vi "OdorSystem-counter-V1.1.vi"() -> ()   [LabVIEW 2019]
doc: "Synchronize Correlated Digital Output with Analog Input Using NI-DAQmx \n\nOverview:\nThis example uses DAQmx to synchronize finite generation and acquisition of Correlated Digital Output with an Analog Input Task respectively.\n\nDescriptions:\nCorrelated I/O enables synchronization of on board digital I/O lines to a clock reference. Digital and Analog samples can be synchronized in time by sharing the AI clock as the source of your digital I/O clock. You may also use the Counter Output pulse as the Source of Digital Timing. Hence, set the Source for Digital Timing as ai/SampleClock.This example will work on any device that uses DAQmx and supports Correlated Digital I/O. To perform Correlated Digital I/O on 9172 Chassis, you need a Correlated Module in slot 1-4 of the chassis. \n\nRequirements:\n1. LabVIEW 2012 or compatible.\n2. NI-DAQmx 15.5.1 or compatible.\n\nInstructions:\n1. Set all the control values on the front panel corresponding to the physical channel to be used on the DAQ device.\n2. Run this VI.\n3. Monitor the analog input voltage measured and ramp signal generated from specified channels. \n\nBlock Diagram Steps:\n1. Creates channels to measure voltage and to generate digital signals \n2. Sets the source of the Sample Clock, the rate of the Sample Clock, and the number of samples to acquire or generate.\n3. Generates an array containing a ramp pattern and write to digital output lines.\n4. Transitions the tasks to running state to begin measuring and generating data.\n5. Reads the waveform from the analog input channel and waits for the digital output generation to complete.\n6. Clears the tasks.\n7. Displays any error occurs."
uses:
  StatesEnum.ctl
  <vilib>/DAQmx/write.llb/DAQmx Write (Digital 1D Bool NChan 1Samp 1Line).vi
  <vilib>/DAQmx/write.llb/DAQmx Write (Digital Wfm 1Chan NSamp).vi
  <vilib>/DAQmx/miscellaneous.llb/DAQmx Fill In Error Info.vi
  <vilib>/DAQmx/create/channels.llb/DAQmx Create Channel (CO-Pulse Generation-Frequency).vi
  <vilib>/Waveform/DWDTOps.llb/Digital Pattern Generator (Single Value).vi
  <vilib>/Waveform/DWDTOps.llb/DWDT Append Digital Samples.vi
  <vilib>/DAQmx/configure/timing.llb/DAQmx Timing (Implicit).vi
  <vilib>/Waveform/DWDTOps.llb/DWDT Append Digital Signals.vi
  <vilib>/Waveform/DWDTOps.llb/DWDT Digital to Boolean Array.vi
  <vilib>/DAQmx/create/channels.llb/DAQmx Create Channel (DO-Digital Output).vi
  <vilib>/DAQmx/configure/timing.llb/DAQmx Timing (Sample Clock).vi
  <vilib>/Waveform/DWDTOps.llb/DWDT Uncompress Digital.vi
panel:
  in  "Use Default vavle":bool=TRUE
  in  "Selected default valve":u8(knob)=8 min=1 max=8 step=1 scale=1.0..8.0
  out "Experiment running":bool
  out "State":T1
  in  "Select experiment":enum32{"Single trial", "Trial series"}(tab)
  out "Time elapsed":dbl format="%.1f"
  in  "Start single trial":bool
  out "single trial done":bool
  in  "Select valve":u8(knob)=1 min=1 max=8 step=1 scale=1.0..8.0
  out "Pause elapsed time":dbl format="%#.1f"
  out "In between trials":bool
  out "Trial elapsed time":dbl format="%.1f"
  out "Total elapsed time":dbl format="%.1f"
  out "Estimated total time":dbl
  out "Current list index":i32
  out "Current Valve":u8
  in  "Time between trials":u16=10 min=1 max=900 step=1
  in  "Start trial series":bool
  in  "Valve order list":i8[](array[numeric]) min=1 max=8 step=1
  out "Digitaler output":digitalwaveform(graph)
  out "Stop Boolesch":bool
  in  "Total trial time":dbl=20.0 min=1.0 step=0.1
  in  "Valve opening Time":dbl=10.0 min=0.0 step=0.1
  in  "Valve delay":dbl=2.0 min=0.0 step=0.1
  in  "Stopp":bool
  out "Digital Waveform Graph":digitalwaveform(graph)
  # "All times are in second!"
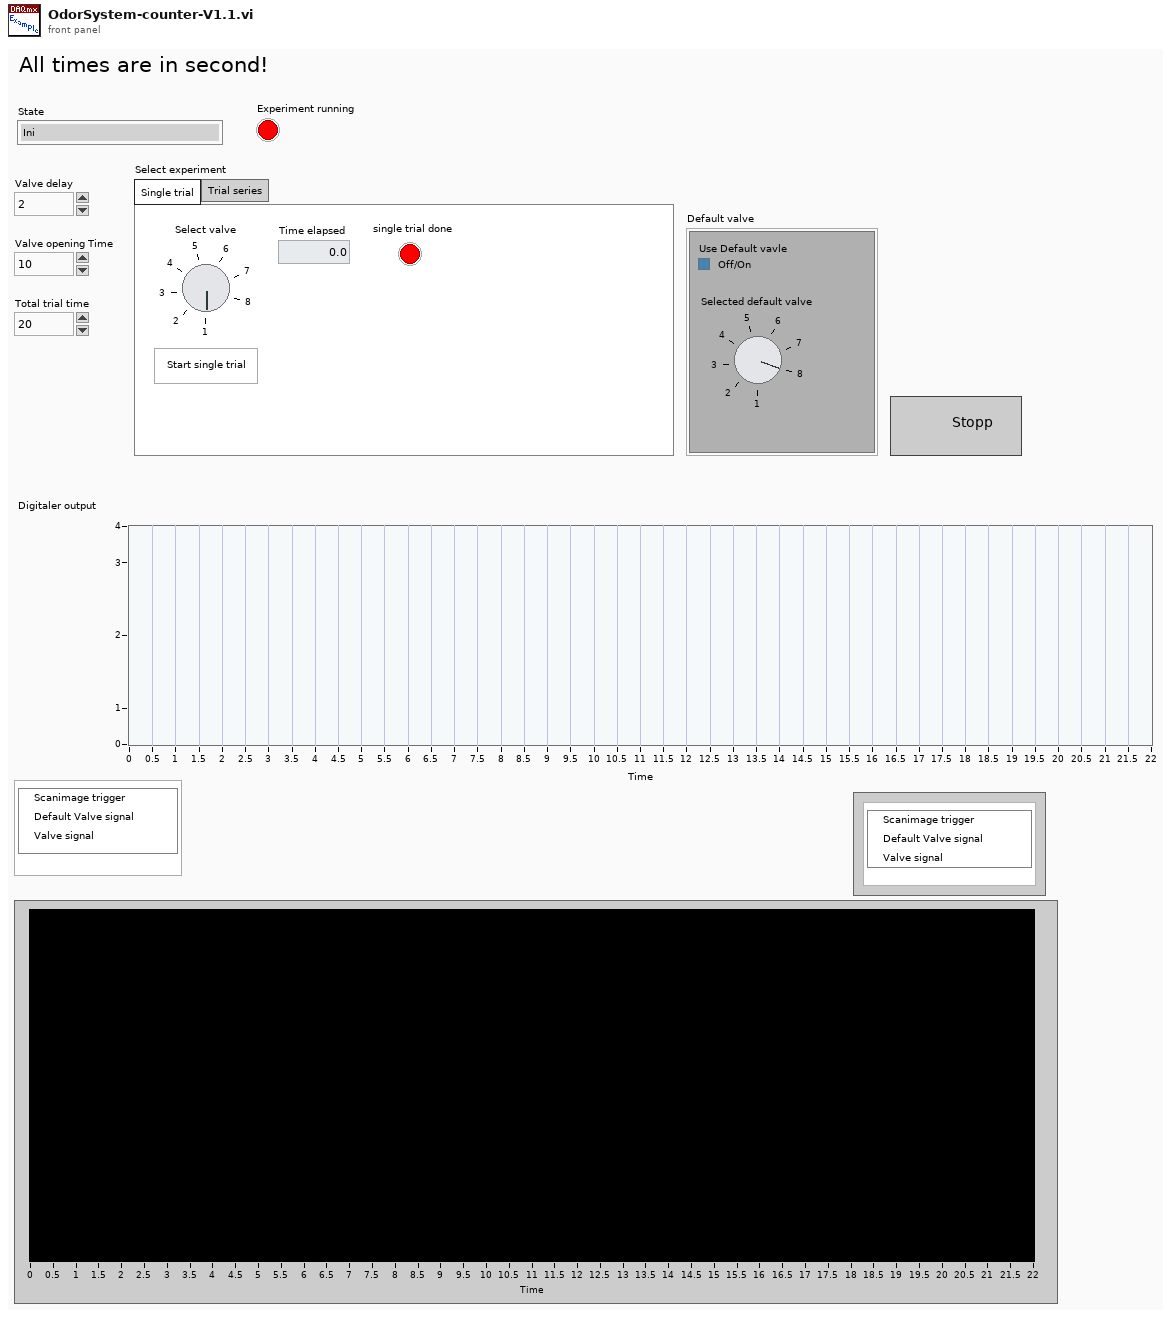
[diagram p1: front panel]
types:
  T1 = typedef "StatesEnum.ctl" = enum16{"Ini", "Standby", "Start Trial", "Start trial series", "Stop"}
  T2 = enum8{"Enabled", "Disabled", "Disabled and Grayed Out"}
  T3 = enum32{"Page Enabled", "Page Disabled", "Page Disabled & Grayed"}
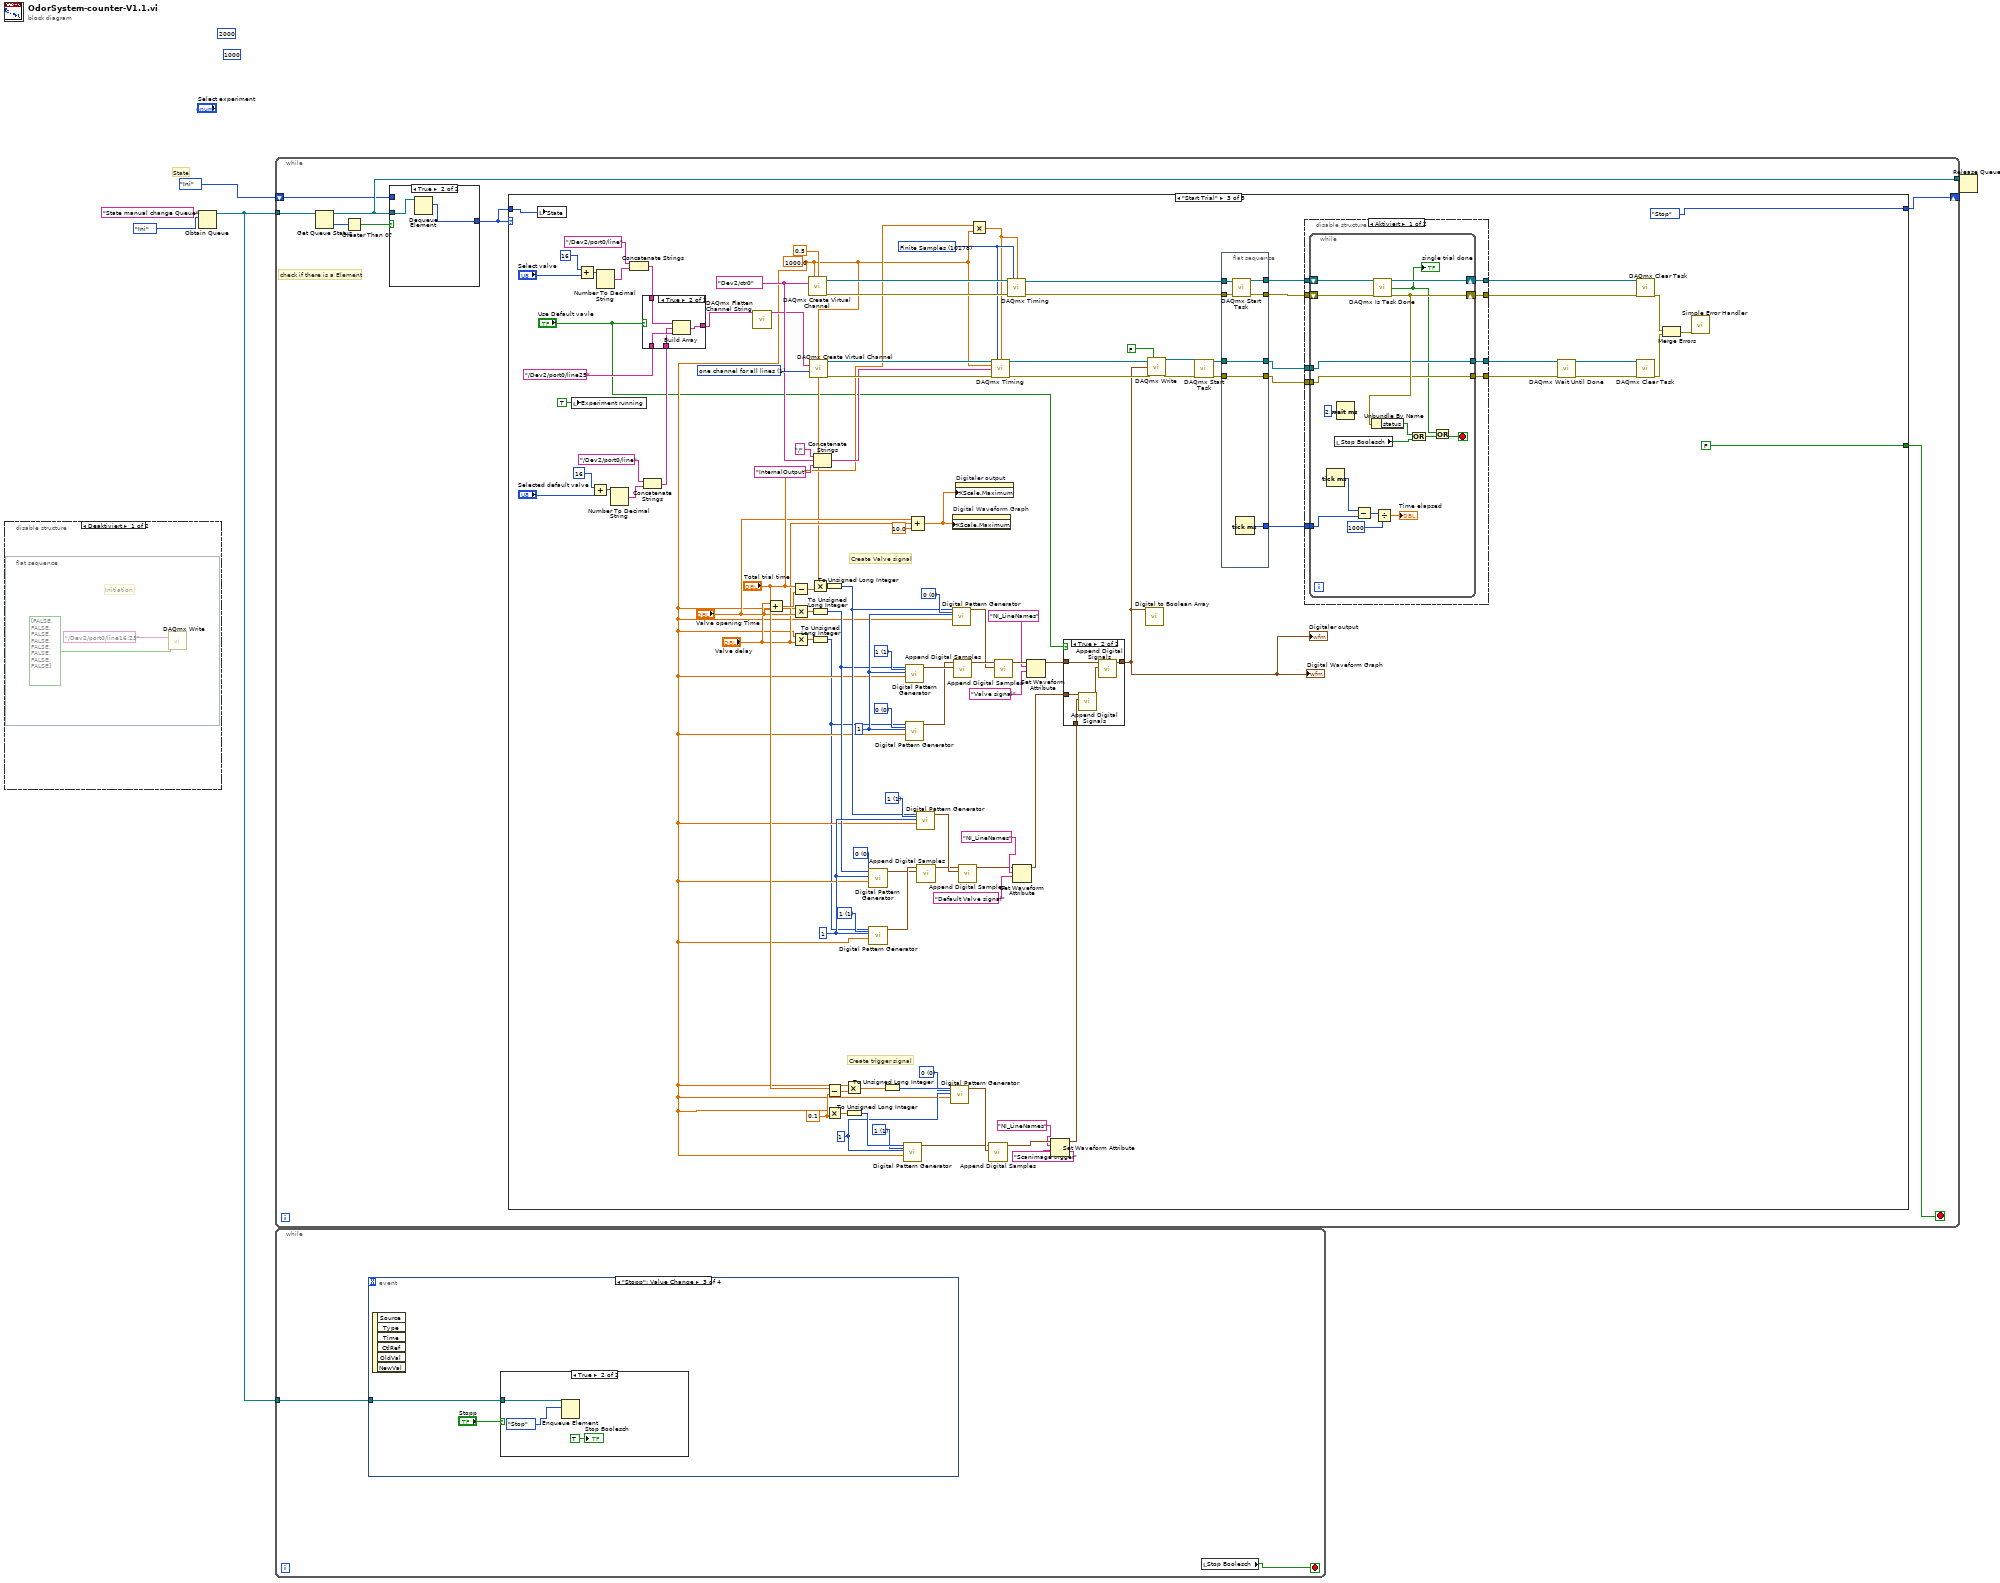
[diagram p0: block diagram]
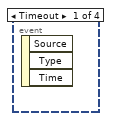
[diagram p3: hidden frame]
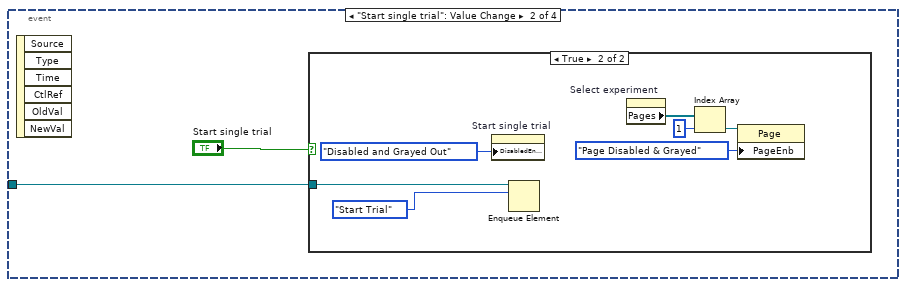
[diagram p4: hidden frame]
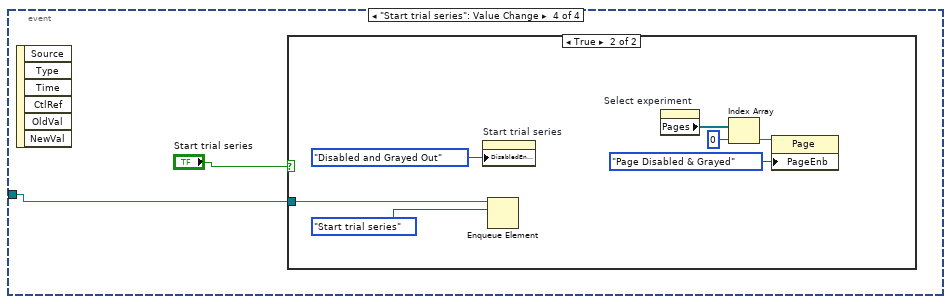
[diagram p7: hidden frame]
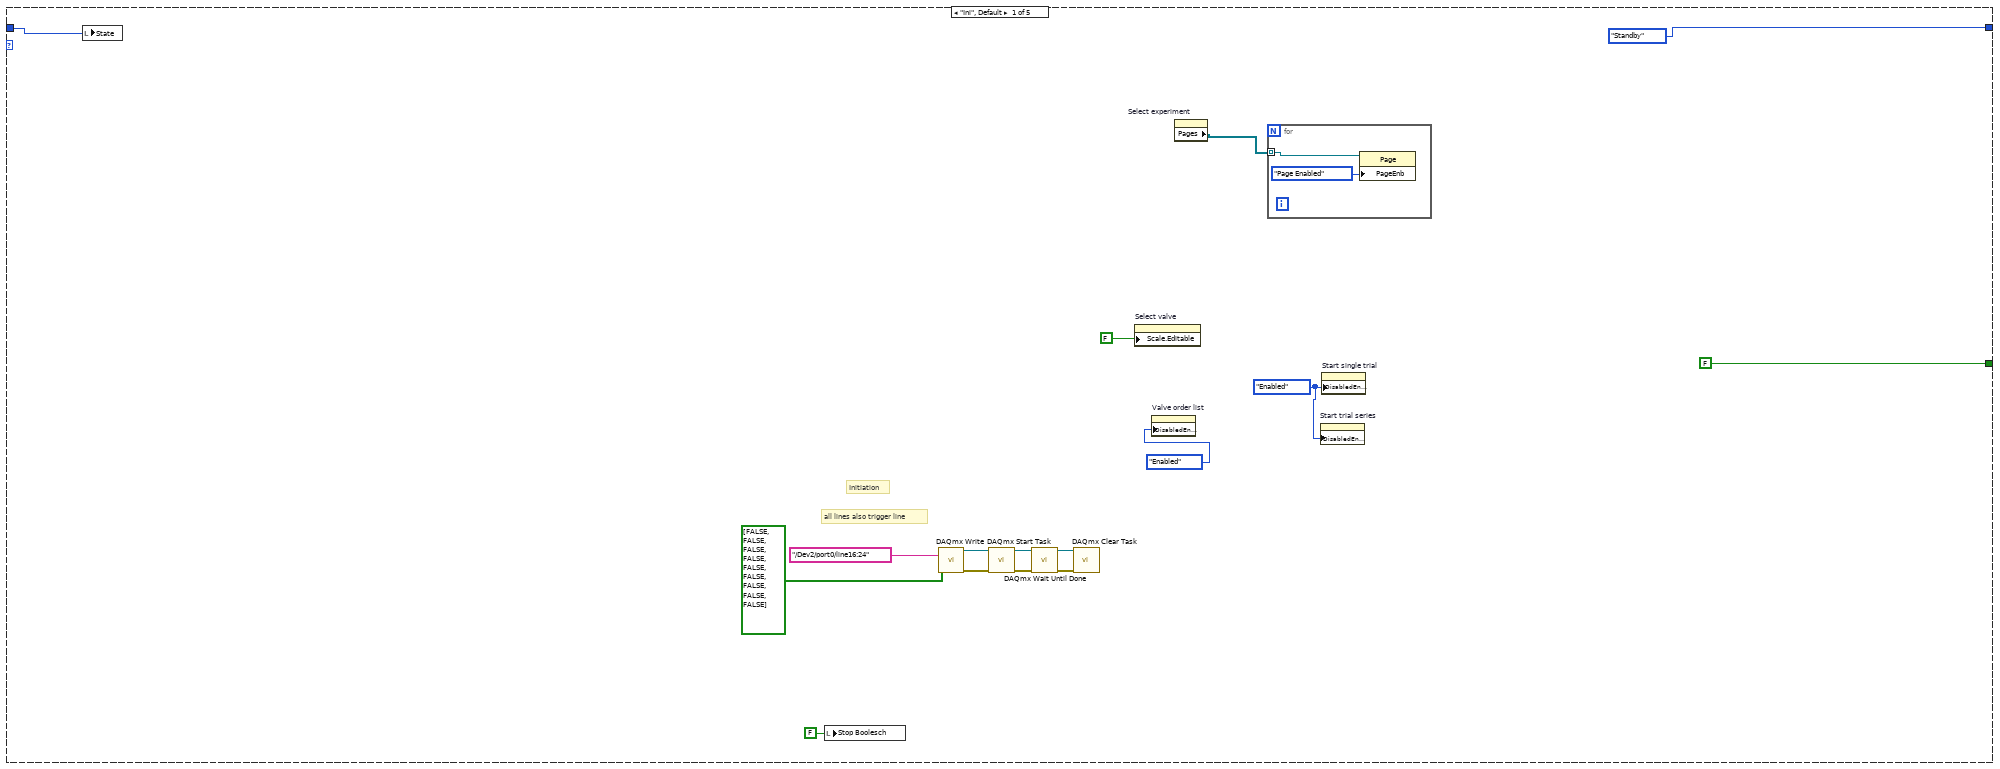
[diagram p10: hidden frame]
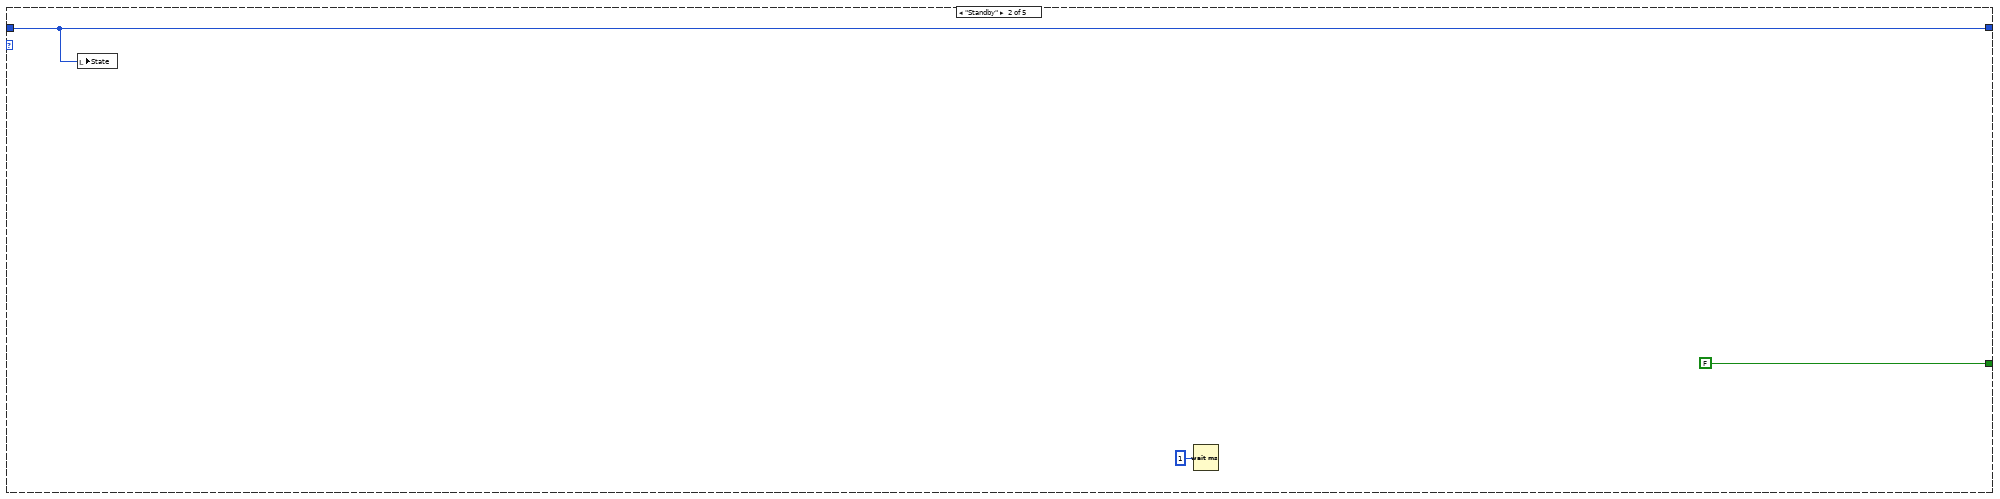
[diagram p11: hidden frame]
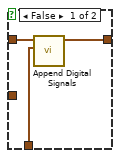
[diagram p12: hidden frame]
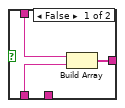
[diagram p13: hidden frame]
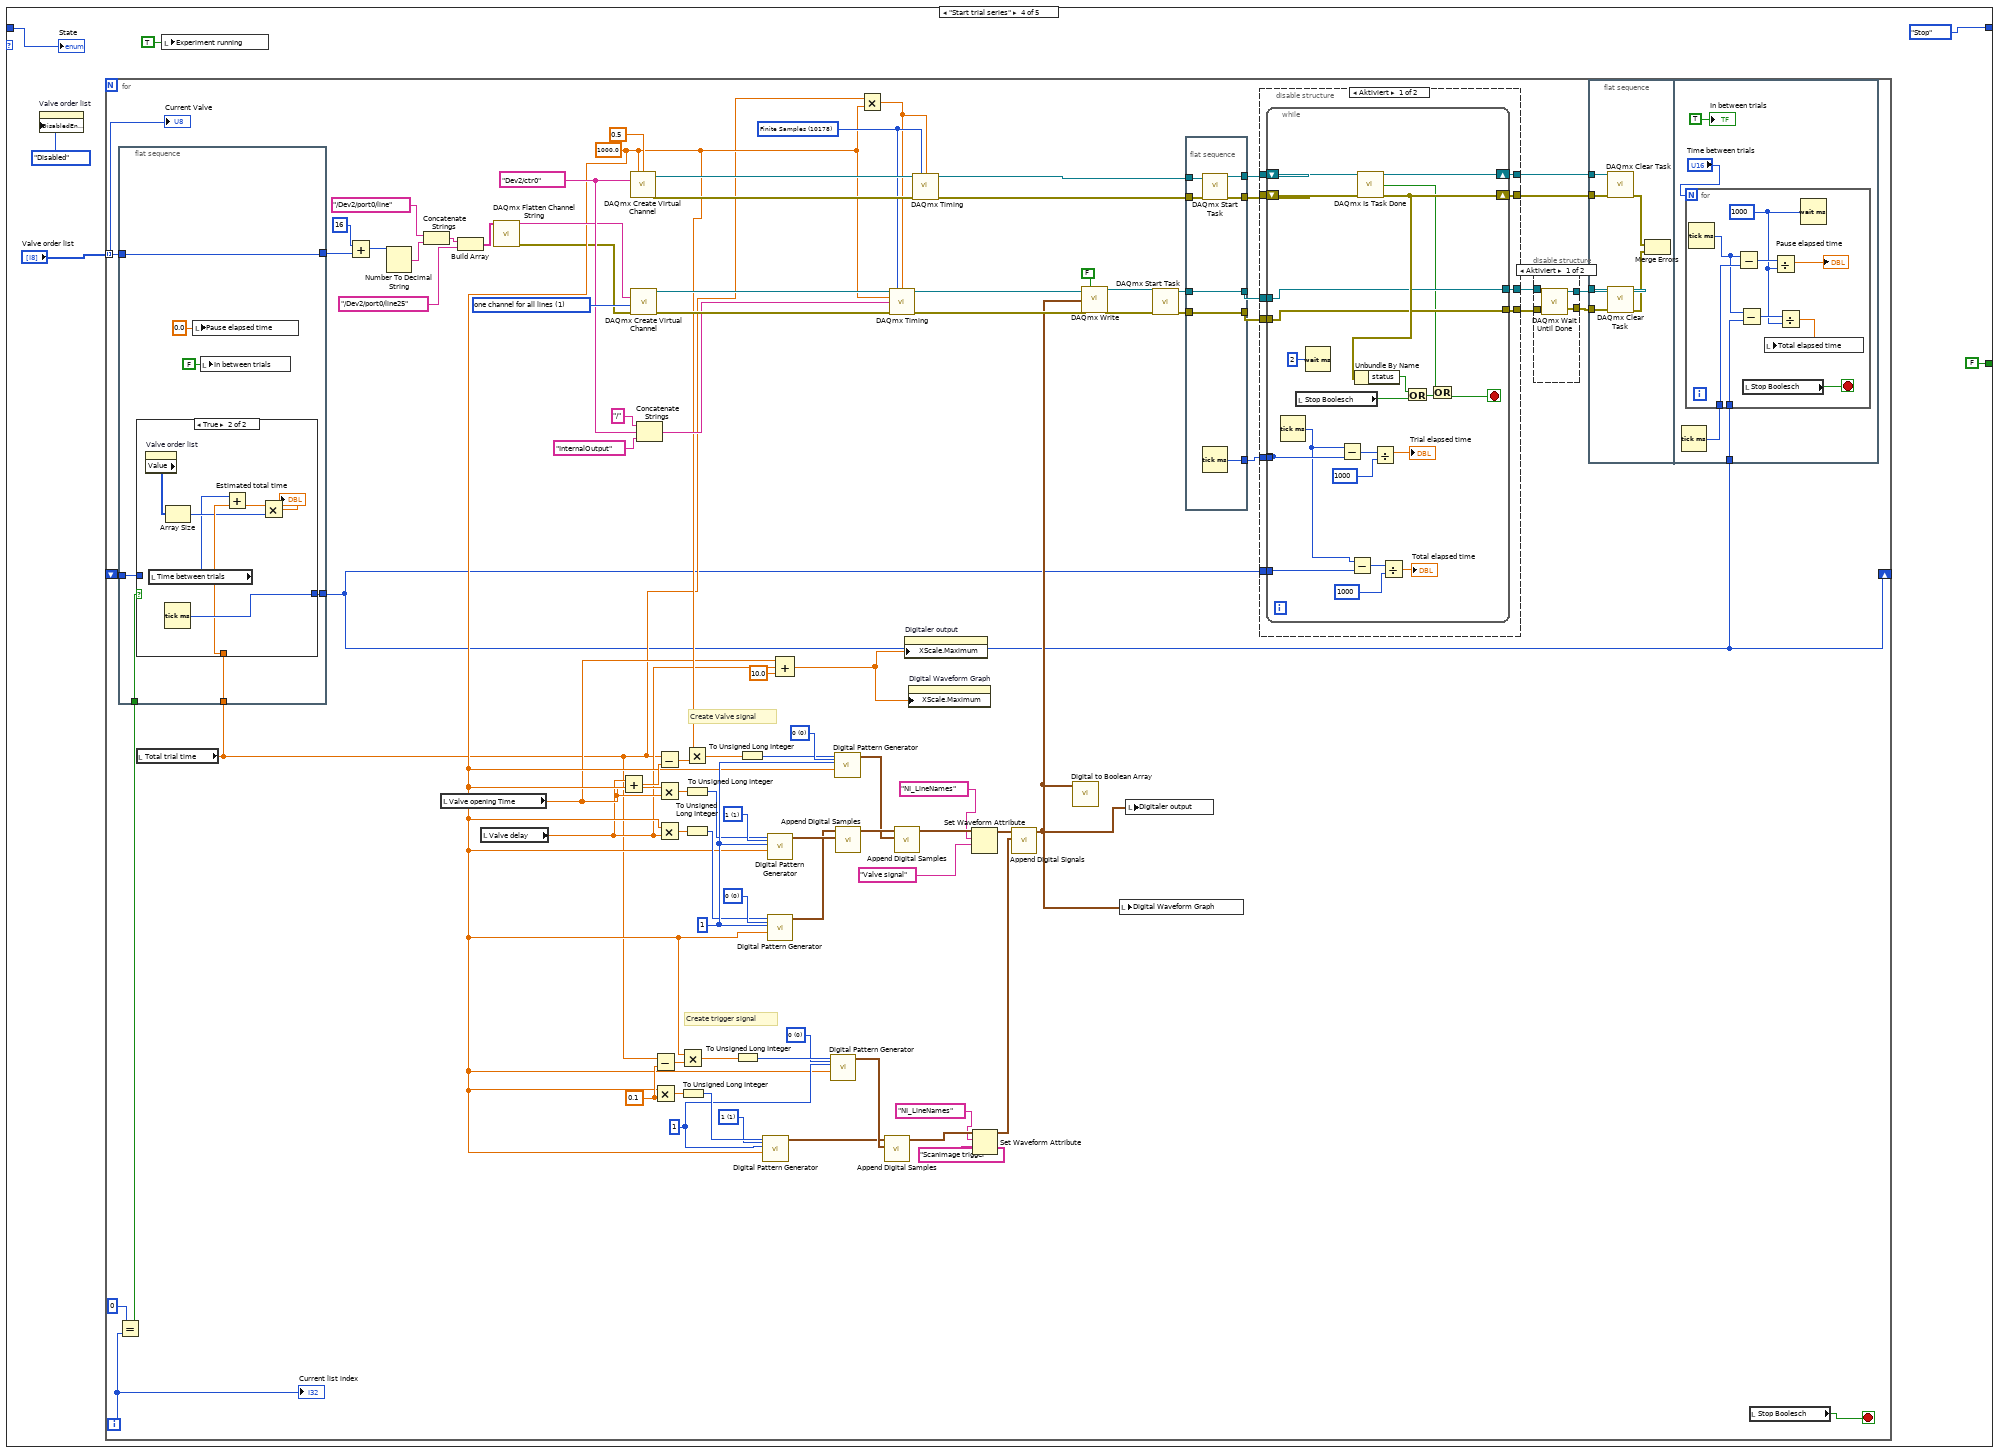
[diagram p15: hidden frame]
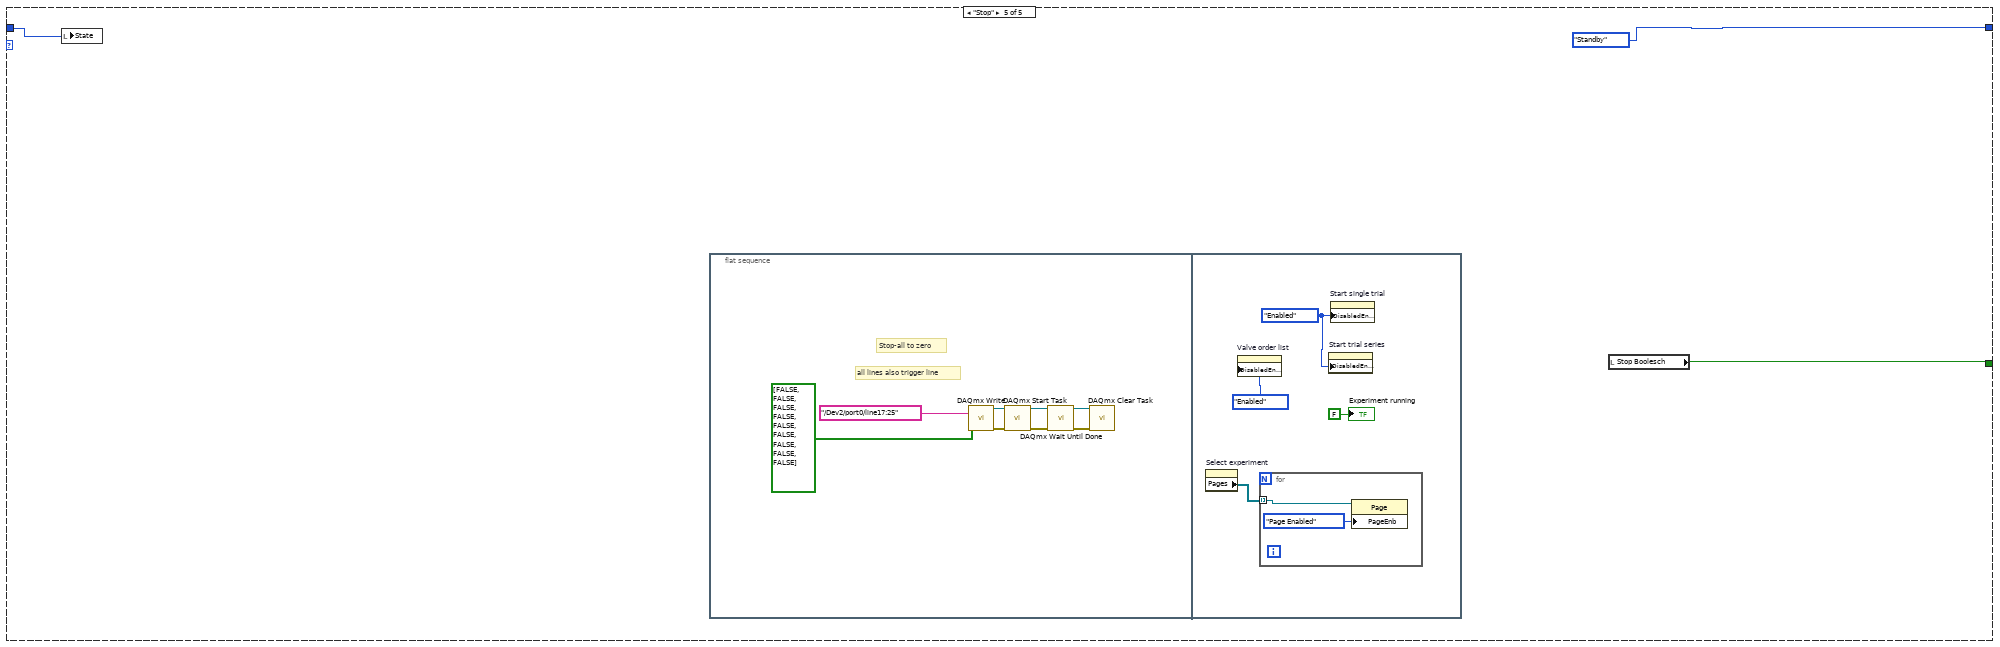
[diagram p19: hidden frame]
diagram:
  (unwired) u32 2000 ("number of samples")
  (unwired) u32 1000 ("number of samples")
  # "State"
  n1 = disable-structure shown="Deaktiviert" {
    frame Disabled {
      n2 = flat-sequence {
        frame #0 {
          # "Initiation"
          n3 = call-poly <vilib>:"DAQmx Write.vi"("task/channels in"="/Dev2/port0/line16:23" ("string"), "data"=bool[] [FALSE, FALSE, FALSE, FALSE, FALSE, FALSE, FALSE, FALSE]) -> ()  [unwired: 11 in, 3 out]
        }
      }
    }
    frame Enabled {
    }
  }
  n4 = Obtain Queue(name (unnamed)="State manual change Queue", element data type=StatesEnum."Ini" ("Enum")) -> (queue out=w4:refnum<queue>)  [unwired: 3 in, 2 out]
  n5 = while {
    tunnel: w4 -> [w13]
    tunnel: [w12] -> w3
    shift-right: [w8] -> _
    shift-left: StatesEnum."Ini" -> [w9]
    stop <- w11 stop-if-true
    # "check if there is a Element"
    n6 = Get Queue Status(queue=w13) -> (queue out=w12:refnum<queue>, # elements in queue=w15:i32)  [unwired: 2 in, 6 out]
    n7 = Greater Than 0?(x=w15) -> (x > 0?=w14:bool)
    n8 = case shown="True" w14 {
      tunnel: w12 -> [_ w18]
      tunnel: w9 -> [w16 _]
      tunnel: [w16 w17] -> w10
      frame False {
      }
      frame True {
        n9 = Dequeue Element(queue=w18) -> (element=w17:T1)  [unwired: 2 in, 3 out]
      }
    }
    n10 = case shown="\"Start Trial\"" w10 {
      tunnel: w10 -> [w29 w37 w66 w199 w369]
      tunnel: [FALSE ("Stop Boolesch") FALSE ("Stop Boolesch") FALSE ("Stop Boolesch") FALSE ("Stop Boolesch") w371] -> w11
      tunnel: [StatesEnum."Standby" ("Enum") w37 StatesEnum."Stop" ("Enum") StatesEnum."Stop" ("Enum") StatesEnum."Standby" ("Enum")] -> w8
      frame "Ini", Default {
        w22 = T2."Enabled" ("Deaktiviert")
        # "all lines also trigger line"
        # "Initiation"
        n11 = local write "State"(w29) -> ()
        n12 = local write "Stop Boolesch"(FALSE ("Stop Boolesch")) -> ()
        n13 = call-poly <vilib>:"DAQmx Write.vi"("task/channels in"="/Dev2/port0/line16:24" ("string"), "data"=bool[] [FALSE, FALSE, FALSE, FALSE, FALSE, FALSE, FALSE, FALSE, FALSE]) -> ("task out"=w24:refnum<k21>, "error out"=w23:errorcluster)  [unwired: 11 in, 1 out]
        n14 = call <vilib>:"DAQmx Start Task.vi"("task/channels in"=w24, "error in"=w23) -> ("task out"=w28:refnum<k21>, "error out"=w26:errorcluster)  [unwired: 12 in]
        n15 = call <vilib>:"DAQmx Wait Until Done.vi"("task/channels in"=w28, "error in"=w26) -> ("task out"=w27:refnum<k21>, "error out"=w25:errorcluster)  [unwired: 12 in]
        n16 = call <vilib>:"DAQmx Clear Task.vi"("task in"=w27, "error in"=w25) -> ()  [unwired: 13 in, 1 out]
        n17 = property on="Select valve" class="Knob (strict)"("Scale.Editable"=FALSE ("Skala.Editierbar")) -> ()  [unwired: 2 in, 2 out]
        n18 = property on="Valve order list" class="Arr (strict)"("DisabledEnum"=T2."Enabled" ("Deaktiviert")) -> ()  [unwired: 2 in, 2 out]
        n19 = property on="Select experiment" class="TabCtl (strict)"() -> ("Pages"=w20:refnum<vi>[])  [unwired: 2 in, 2 out]
        n20 = for {
          tunnel: w20 -> [w35] mode=indexing
          n21 = property class="Page"(reference=w35, "PageEnb"=T3."Page Enabled" ("Aktiv-Status der Seite")) -> ()  [unwired: 1 in, 2 out]
        }
        n22 = property on="Start trial series" class="Bool"("DisabledEnum"=w22) -> ()  [unwired: 2 in, 2 out]
        n23 = property on="Start single trial" class="Bool"("DisabledEnum"=w22) -> ()  [unwired: 2 in, 2 out]
      }
      frame "Standby" {
        n24 = local write "State"(w37) -> ()
        n25 = Wait (ms)(milliseconds to wait=u32 1 ("Zu wartende ms")) -> ()  [unwired: 1 out]
      }
      frame "Start Trial" {
        w52 = u32 1 ("number of signals")
        w55 = u8 1 items=["0", "1", "Z", "L", "H", "X", "T", "V"] ("value")
        w54 = u8 0 items=["0", "1", "Z", "L", "H", "X", "T", "V"] ("value")
        w53 = u8 1 items=["0", "1", "Z", "L", "H", "X", "T", "V"] ("value")
        w89 = 0.1 ("y")
        w96 = u32 1 ("number of signals")
        w98 = u8 0 items=["0", "1", "Z", "L", "H", "X", "T", "V"] ("value")
        w97 = u8 1 items=["0", "1", "Z", "L", "H", "X", "T", "V"] ("value")
        w114 = tag "Dev2/ctr0" ("counter")
        w49 = 1000.0 ("frequency")
        w123 = u32 1 ("number of signals")
        w124 = u8 0 items=["0", "1", "Z", "L", "H", "X", "T", "V"] ("value")
        w125 = u8 1 items=["0", "1", "Z", "L", "H", "X", "T", "V"] ("value")
        w126 = u8 0 items=["0", "1", "Z", "L", "H", "X", "T", "V"] ("value")
        w137 = 1 items=["one channel for each line", "one channel for all lines"] ("line grouping")
        w118 = 10178 items=["Finite Samples"=10178, "Continuous Samples"=10123] ("sample mode")
        # "Create trigger signal"
        # "Create Valve signal"
        n26 = local write "State"(w66) -> ()
        n27 = local write "Experiment running"(TRUE ("Experiment running")) -> ()
        n28 = Add(x=i8 16, y="Select valve") -> (x+y=w105:u8)
        n29 = Add(x=i8 16, y="Selected default valve") -> (x+y=w46:u8)
        n30 = Number To Decimal String(number=w105) -> (decimal integer string=w106:string)  [unwired: 1 in]
        n31 = Number To Decimal String(number=w46) -> (decimal integer string=w45:string)  [unwired: 1 in]
        n32 = Concatenate Strings("/Dev2/port0/line" ("string"), w106) -> (w95:string)
        n33 = Concatenate Strings("/Dev2/port0/line" ("string"), w45) -> (w43:string)
        n34 = case shown="True" "Use Default vavle" {
          tunnel: w95 -> [w158 w161]
          tunnel: "/Dev2/port0/line25" ("string") -> [w157 w160]
          tunnel: [w156 w162] -> w93
          tunnel: w43 -> [_ w159]
          frame False {
            n35 = Build Array(w158, w157) -> (w156:string[])
          }
          frame True {
            n36 = Build Array(w161, w159, w160) -> (w162:string[])
          }
        }
        n37 = call <vilib>:"DAQmx Flatten Channel String.vi"("names in"=w93) -> ("names out"=w92:string)  [unwired: 13 in, 1 out]
        n38 = Add(x="Valve delay", y="Valve opening Time") -> (x+y=w109:dbl)
        n39 = Subtract(x="Total trial time", y=w109) -> (x-y=w108:dbl)
        n40 = Multiply(x=w49, y="Valve opening Time") -> (x*y=w111:dbl)
        n41 = Multiply(x=w49, y="Valve delay") -> (x*y=w112:dbl)
        n42 = call-poly <vilib>:"DAQmx Create Virtual Channel.vi"("frequency"=w49, "duty cycle"=0.5, "counter"=w114) -> ("task out"=w142:refnum<k21>, "error out"=w143:errorcluster)  [unwired: 11 in]
        n43 = call-poly <vilib>:"DAQmx Create Virtual Channel.vi"("lines"=w92, "line grouping"=w137) -> ("task out"=w147:refnum<k21>, "error out"=w146:errorcluster)  [unwired: 12 in]
        n44 = Multiply(x=w49, y=w108) -> (x*y=w110:dbl)
        n45 = To Unsigned Long Integer(number=w111) -> (unsigned 32bit integer=w50:u32)
        n46 = To Unsigned Long Integer(number=w112) -> (unsigned 32bit integer=w48:u32)
        n47 = Concatenate Strings("/", w114, "InternalOutput" ("string")) -> (w113:string)
        n48 = To Unsigned Long Integer(number=w110) -> (unsigned 32bit integer=w51:u32)
        n49 = Subtract(x="Total trial time", y=w89) -> (x-y=w103:dbl)
        n50 = Multiply(x=w49, y=w89) -> (x*y=w99:dbl)
        n51 = Multiply(x=w49, y=w103) -> (x*y=w101:dbl)
        n52 = To Unsigned Long Integer(number=w99) -> (unsigned 32bit integer=w100:u32)
        n53 = call-poly <vilib>:"Digital Pattern Generator.vi"("value"=w54, "sample rate"=w49, "number of signals"=w52, "number of samples"=w50) -> ("digital waveform"=w59:digitalwaveform)  [unwired: 6 in, 1 out]
        n54 = call-poly <vilib>:"Digital Pattern Generator.vi"("value"=w53, "sample rate"=w49, "number of signals"=w52, "number of samples"=w48) -> ("digital waveform"=w60:digitalwaveform)  [unwired: 6 in, 1 out]
        n55 = To Unsigned Long Integer(number=w101) -> (unsigned 32bit integer=w102:u32)
        n56 = call-poly <vilib>:"Digital Pattern Generator.vi"("value"=w97, "sample rate"=w49, "number of signals"=w96, "number of samples"=w100) -> ("digital waveform"=w77:digitalwaveform)  [unwired: 6 in, 1 out]
        n57 = call-poly <vilib>:"Digital Pattern Generator.vi"("value"=w125, "sample rate"=w49, "number of signals"=w123, "number of samples"=w50) -> ("digital waveform"=w82:digitalwaveform)  [unwired: 6 in, 1 out]
        n58 = call-poly <vilib>:"Digital Pattern Generator.vi"("value"=w126, "sample rate"=w49, "number of signals"=w123, "number of samples"=w48) -> ("digital waveform"=w81:digitalwaveform)  [unwired: 6 in, 1 out]
        n59 = Compound Arithmetic op=ADD("Valve opening Time", "Valve delay", 10.0 ("Wert")) -> (w67:dbl)
        n60 = call-poly <vilib>:"Digital Pattern Generator.vi"("value"=w55, "sample rate"=w49, "number of signals"=w52, "number of samples"=w51) -> ("digital waveform"=w62:digitalwaveform)  [unwired: 6 in, 1 out]
        n61 = call-poly <vilib>:"Append Digital Samples.vi"("digital waveform B"=w59, "digital waveform A"=w60) -> ("digital waveform out"=w61:digitalwaveform)  [unwired: 8 in, 1 out]
        n62 = call-poly <vilib>:"Digital Pattern Generator.vi"("value"=w98, "sample rate"=w49, "number of signals"=w96, "number of samples"=w102) -> ("digital waveform"=w78:digitalwaveform)  [unwired: 6 in, 1 out]
        n63 = property on="Digital Waveform Graph" class="DigitalGraph (strict)"("XScale.Maximum"=w67) -> ()  [unwired: 2 in, 2 out]
        n64 = call-poly <vilib>:"Digital Pattern Generator.vi"("value"=w124, "sample rate"=w49, "number of signals"=w123, "number of samples"=w51) -> ("digital waveform"=w79:digitalwaveform)  [unwired: 6 in, 1 out]
        n65 = call-poly <vilib>:"Append Digital Samples.vi"("digital waveform B"=w82, "digital waveform A"=w81) -> ("digital waveform out"=w80:digitalwaveform)  [unwired: 8 in, 1 out]
        n66 = property on="Digitaler output" class="DigitalGraph (strict)"("XScale.Maximum"=w67) -> ()  [unwired: 2 in, 2 out]
        n67 = call-poly <vilib>:"Append Digital Samples.vi"("digital waveform B"=w62, "digital waveform A"=w61) -> ("digital waveform out"=w56:digitalwaveform)  [unwired: 8 in, 1 out]
        n68 = Multiply(x="Total trial time", y=w49) -> (x*y=w90:dbl)
        n69 = call-poly <vilib>:"Append Digital Samples.vi"("digital waveform B"=w78, "digital waveform A"=w77) -> ("digital waveform out"=w88:digitalwaveform)  [unwired: 8 in, 1 out]
        n70 = call-poly <vilib>:"DAQmx Timing.vi"("task/channels in"=w147, "sample mode"=w118, "samples per channel"=w90, "rate"=w49, "source"=w113, "error in"=w146) -> ("task out"=w134:refnum<k21>, "error out"=w133:errorcluster)  [unwired: 8 in]
        n71 = call-poly <vilib>:"Append Digital Samples.vi"("digital waveform B"=w79, "digital waveform A"=w80) -> ("digital waveform out"=w85:digitalwaveform)  [unwired: 8 in, 1 out]
        n72 = call-poly <vilib>:"DAQmx Timing.vi"("task/channels in"=w142, "sample mode"=w118, "samples per channel"=w90, "error in"=w143) -> ("task out"=w140:refnum<k21>, "error out"=w141:errorcluster)  [unwired: 10 in]
        n73 = Set Waveform Attribute(5:"Default Valve signal", 6:"NI_LineNames" ("name"), 7:w56) -> (3:w40:digitalwaveform)  [unwired: 1 in, 2 out]
        n74 = Set Waveform Attribute(5:"Valve signal", 6:"NI_LineNames" ("name"), 7:w85) -> (3:w76:digitalwaveform)  [unwired: 1 in, 2 out]
        n75 = Set Waveform Attribute(5:"Scanimage trigger", 6:"NI_LineNames" ("name"), 7:w88) -> (3:w75:digitalwaveform)  [unwired: 1 in, 2 out]
        n76 = case shown="True" "Use Default vavle" {
          tunnel: w76 -> [w150 w155]
          tunnel: w75 -> [w149 w153]
          tunnel: [w148 w154] -> w69
          tunnel: w40 -> [_ w152]
          frame False {
            n77 = call-poly <vilib>:"Append Digital Signals.vi"("digital waveform (low bits)"=w149, "digital waveform (high bits)"=w150) -> ("digital waveform out"=w148:digitalwaveform)  [unwired: 8 in, 1 out]
          }
          frame True {
            n78 = call-poly <vilib>:"Append Digital Signals.vi"("digital waveform (low bits)"=w153, "digital waveform (high bits)"=w152) -> ("digital waveform out"=w151:digitalwaveform)  [unwired: 8 in, 1 out]
            n79 = call-poly <vilib>:"Append Digital Signals.vi"("digital waveform (low bits)"=w151, "digital waveform (high bits)"=w155) -> ("digital waveform out"=w154:digitalwaveform)  [unwired: 8 in, 1 out]
          }
        }
        "Digital Waveform Graph" <- w69
        "Digitaler output" <- w69
        n80 = call-poly <vilib>:"Digital to Boolean Array.vi"("digital waveform"=w69) -> ()  [unwired: 9 in, 2 out]
        n81 = call-poly <vilib>:"DAQmx Write.vi"("task/channels in"=w134, "auto start"=FALSE, "data"=w69, "error in"=w133) -> ("task out"=w132:refnum<k21>, "error out"=w131:errorcluster)  [unwired: 9 in, 1 out]
        n82 = call <vilib>:"DAQmx Start Task.vi"("task/channels in"=w132, "error in"=w131) -> ("task out"=w136:refnum<k21>, "error out"=w135:errorcluster)  [unwired: 12 in]
        n83 = flat-sequence {
          tunnel: [w195] -> w145
          tunnel: [w194] -> w144
          tunnel: w141 -> [w193]
          tunnel: w140 -> [w192]
          tunnel: [w191] -> w122
          tunnel: w136 -> [w191]
          tunnel: [w190] -> w121
          tunnel: w135 -> [w190]
          tunnel: [w189] -> w64
          frame #0 {
            n84 = call <vilib>:"DAQmx Start Task.vi"("task/channels in"=w192, "error in"=w193) -> ("task out"=w195:refnum<k21>, "error out"=w194:errorcluster)  [unwired: 12 in]
            n85 = Tick Count (ms)() -> (millisecond timer value=w189:u32)
          }
        }
        n86 = disable-structure shown="Aktiviert" {
          disable-tunnel: w145 -> [w171 _]
          disable-tunnel: w144 -> [w170 _]
          disable-tunnel: [w169 _] -> w139
          disable-tunnel: [w168 _] -> w138
          disable-tunnel: w122 -> [w167 _]
          disable-tunnel: w121 -> [w166 _]
          disable-tunnel: [w165 _] -> w120
          disable-tunnel: [w164 _] -> w119
          disable-tunnel: w64 -> [w163 _]
          frame Enabled {
            n87 = while {
              shift-right: [w185] -> w168
              shift-left: w171 -> [w187]
              shift-right: [w184] -> w169
              shift-left: w170 -> [w186]
              tunnel: w167 -> [w183]
              tunnel: w166 -> [w182]
              tunnel: [w183] -> w165
              tunnel: [w182] -> w164
              tunnel: w163 -> [w175]
              stop <- w178 stop-if-true
              n88 = Tick Count (ms)() -> (millisecond timer value=w176:u32)
              n89 = local read "Stop Boolesch"() -> (w179:bool)
              n90 = Wait (ms)(milliseconds to wait=u32 2 ("Zu wartende ms")) -> ()  [unwired: 1 out]
              n91 = Subtract(x=w176, y=w175) -> (x-y=w174:u32)
              n92 = call <vilib>:"DAQmx Is Task Done.vi"("task/channels in"=w187, "error in"=w186) -> ("task out"=w185:refnum<k21>, "task done?"=w177:bool, "error out"=w184:errorcluster)  [unwired: 11 in]
              "single trial done" <- w177
              n93 = Unbundle By Name(w184) -> ("status"=w180:bool)
              n94 = Divide(x=w174, y=u32 1000) -> (x/y=→"Time elapsed":dbl)
              n95 = Or(x=w180, y=w179) -> (x .or. y?=w188:bool)
              n96 = Or(x=w177, y=w188) -> (x .or. y?=w178:bool)
            }
          }
          frame Disabled {
          }
        }
        n97 = call <vilib>:"DAQmx Wait Until Done.vi"("task/channels in"=w120) -> ("task out"=w71:refnum<k21>)  [unwired: 13 in, 1 out]
        n98 = call <vilib>:"DAQmx Clear Task.vi"("task in"=w138, "error in"=w139) -> ("error out"=w129:errorcluster)  [unwired: 13 in]
        n99 = call <vilib>:"DAQmx Clear Task.vi"("task in"=w71, "error in"=w119) -> ("error out"=w128:errorcluster)  [unwired: 13 in]
        n100 = Merge Errors(w129, w128) -> (w127:errorcluster)
        n101 = call <vilib>:"Simple Error Handler.vi"("error in (no error)"=w127) -> ()  [unwired: 4 in, 5 out]
      }
      frame "Start trial series" {
        n102 = property on="Valve order list" class="Arr (strict)"("DisabledEnum"=T2."Disabled" ("Deaktiviert")) -> ()  [unwired: 2 in, 2 out]
        n103 = for {
          tunnel: "Valve order list" -> [w207] mode=indexing
          shift-right: [w203] -> _
          shift-left: _ -> [w205]
          i -> [w213]
          stop <- w217 stop-if-true
          w238 = 0.1 ("y")
          w244 = u32 1 ("number of signals")
          w246 = u8 0 items=["0", "1", "Z", "L", "H", "X", "T", "V"] ("value")
          w245 = u8 1 items=["0", "1", "Z", "L", "H", "X", "T", "V"] ("value")
          w265 = tag "Dev2/ctr0" ("counter")
          w222 = 1000.0 ("frequency")
          w273 = u32 1 ("number of signals")
          w274 = u8 0 items=["0", "1", "Z", "L", "H", "X", "T", "V"] ("value")
          w275 = u8 1 items=["0", "1", "Z", "L", "H", "X", "T", "V"] ("value")
          w276 = u8 0 items=["0", "1", "Z", "L", "H", "X", "T", "V"] ("value")
          w284 = 1 items=["one channel for each line", "one channel for all lines"] ("line grouping")
          w269 = 10178 items=["Finite Samples"=10178, "Continuous Samples"=10123] ("sample mode")
          # "Create trigger signal"
          # "Create Valve signal"
          n104 = Equal?(x=0, y=w213) -> (x = y?=w206:bool)
          n105 = flat-sequence {
            tunnel: [w303] -> w208
            tunnel: w207 -> [w303]
            tunnel: w206 -> [w302]
            tunnel: w205 -> [w301]
            tunnel: w204 -> [w300]
            tunnel: [w299] -> w203
            frame #0 {
              n106 = case shown="True" w302 {
                tunnel: [w304 w311] -> w299
                tunnel: w301 -> [w304 _]
                tunnel: w300 -> [_ w310]
                frame False {
                }
                frame True {
                  n107 = property on="Valve order list" class="Arr (strict)"() -> ("Value"=w308:i8[])  [unwired: 2 in, 2 out]
                  n108 = local read "Time between trials"() -> (w305:u16)
                  n109 = Tick Count (ms)() -> (millisecond timer value=w311:u32)
                  n110 = Array Size(array=w308) -> (size(s)=w307:i32)
                  n111 = Add(x=w305, y=w310) -> (x+y=w306:dbl)
                  n112 = Multiply(x=w306, y=w307) -> (x*y=→"Estimated total time":dbl)
                }
              }
              n113 = local write "Pause elapsed time"(0.0 ("Pause elapsed time")) -> ()
              n114 = local write "In between trials"(FALSE ("In between trials")) -> ()
            }
          }
          n115 = local read "Total trial time"() -> (w204:dbl)
          n116 = Add(x=i8 16, y=w208) -> (x+y=w253:i8)
          n117 = Number To Decimal String(number=w253) -> (decimal integer string=w254:string)  [unwired: 1 in]
          n118 = Concatenate Strings("/Dev2/port0/line" ("string"), w254) -> (w243:string)
          n119 = local read "Valve opening Time"() -> (w219:dbl)
          n120 = Build Array(w243, "/Dev2/port0/line25" ("string")) -> (w241:string[])
          n121 = local read "Valve delay"() -> (w218:dbl)
          n122 = call <vilib>:"DAQmx Flatten Channel String.vi"("names in"=w241) -> ("names out"=w240:string, "error out"=w202:errorcluster)  [unwired: 13 in]
          n123 = Add(x=w218, y=w219) -> (x+y=w257:dbl)
          n124 = call-poly <vilib>:"DAQmx Create Virtual Channel.vi"("frequency"=w222, "duty cycle"=0.5, "counter"=w265) -> ("task out"=w287:refnum<k21>, "error out"=w288:errorcluster)  [unwired: 11 in]
          n125 = call-poly <vilib>:"DAQmx Create Virtual Channel.vi"("lines"=w240, "line grouping"=w284, "error in"=w202) -> ("task out"=w292:refnum<k21>, "error out"=w291:errorcluster)  [unwired: 11 in]
          n126 = Concatenate Strings("/", w265, "InternalOutput" ("string")) -> (w264:string)
          n127 = Subtract(x=w204, y=w238) -> (x-y=w251:dbl)
          n128 = Multiply(x=w222, y=w238) -> (x*y=w247:dbl)
          n129 = Subtract(x=w204, y=w257) -> (x-y=w256:dbl)
          n130 = Multiply(x=w222, y=w219) -> (x*y=w261:dbl)
          n131 = Multiply(x=w222, y=w218) -> (x*y=w263:dbl)
          n132 = Multiply(x=w222, y=w251) -> (x*y=w249:dbl)
          n133 = To Unsigned Long Integer(number=w247) -> (unsigned 32bit integer=w248:u32)
          n134 = Multiply(x=w222, y=w256) -> (x*y=w259:dbl)
          n135 = To Unsigned Long Integer(number=w261) -> (unsigned 32bit integer=w260:u32)
          n136 = To Unsigned Long Integer(number=w263) -> (unsigned 32bit integer=w262:u32)
          n137 = To Unsigned Long Integer(number=w249) -> (unsigned 32bit integer=w250:u32)
          n138 = To Unsigned Long Integer(number=w259) -> (unsigned 32bit integer=w258:u32)
          n139 = call-poly <vilib>:"Digital Pattern Generator.vi"("value"=w245, "sample rate"=w222, "number of signals"=w244, "number of samples"=w248) -> ("digital waveform"=w226:digitalwaveform)  [unwired: 6 in, 1 out]
          n140 = call-poly <vilib>:"Digital Pattern Generator.vi"("value"=w275, "sample rate"=w222, "number of signals"=w273, "number of samples"=w260) -> ("digital waveform"=w231:digitalwaveform)  [unwired: 6 in, 1 out]
          n141 = call-poly <vilib>:"Digital Pattern Generator.vi"("value"=w276, "sample rate"=w222, "number of signals"=w273, "number of samples"=w262) -> ("digital waveform"=w230:digitalwaveform)  [unwired: 6 in, 1 out]
          n142 = Compound Arithmetic op=ADD(w219, w218, 10.0 ("Wert")) -> (w220:dbl)
          n143 = call-poly <vilib>:"Digital Pattern Generator.vi"("value"=w246, "sample rate"=w222, "number of signals"=w244, "number of samples"=w250) -> ("digital waveform"=w227:digitalwaveform)  [unwired: 6 in, 1 out]
          n144 = call-poly <vilib>:"Digital Pattern Generator.vi"("value"=w274, "sample rate"=w222, "number of signals"=w273, "number of samples"=w258) -> ("digital waveform"=w228:digitalwaveform)  [unwired: 6 in, 1 out]
          n145 = call-poly <vilib>:"Append Digital Samples.vi"("digital waveform B"=w231, "digital waveform A"=w230) -> ("digital waveform out"=w229:digitalwaveform)  [unwired: 8 in, 1 out]
          n146 = Multiply(x=w204, y=w222) -> (x*y=w239:dbl)
          n147 = call-poly <vilib>:"Append Digital Samples.vi"("digital waveform B"=w227, "digital waveform A"=w226) -> ("digital waveform out"=w237:digitalwaveform)  [unwired: 8 in, 1 out]
          n148 = call-poly <vilib>:"DAQmx Timing.vi"("task/channels in"=w292, "sample mode"=w269, "samples per channel"=w239, "rate"=w222, "source"=w264, "error in"=w291) -> ("task out"=w281:refnum<k21>, "error out"=w280:errorcluster)  [unwired: 8 in]
          n149 = call-poly <vilib>:"Append Digital Samples.vi"("digital waveform B"=w228, "digital waveform A"=w229) -> ("digital waveform out"=w234:digitalwaveform)  [unwired: 8 in, 1 out]
          n150 = property on="Digitaler output" class="DigitalGraph (strict)"("XScale.Maximum"=w220) -> ()  [unwired: 2 in, 2 out]
          n151 = property on="Digital Waveform Graph" class="DigitalGraph (strict)"("XScale.Maximum"=w220) -> ()  [unwired: 2 in, 2 out]
          n152 = call-poly <vilib>:"DAQmx Timing.vi"("task/channels in"=w287, "sample mode"=w269, "samples per channel"=w239, "error in"=w288) -> ("task out"=w285:refnum<k21>, "error out"=w286:errorcluster)  [unwired: 10 in]
          n153 = Set Waveform Attribute(5:"Valve signal", 6:"NI_LineNames" ("name"), 7:w234) -> (3:w225:digitalwaveform)  [unwired: 1 in, 2 out]
          n154 = Set Waveform Attribute(5:"Scanimage trigger", 6:"NI_LineNames" ("name"), 7:w237) -> (3:w224:digitalwaveform)  [unwired: 1 in, 2 out]
          n155 = call-poly <vilib>:"Append Digital Signals.vi"("digital waveform (low bits)"=w224, "digital waveform (high bits)"=w225) -> ("digital waveform out"=w221:digitalwaveform)  [unwired: 8 in, 1 out]
          n156 = call-poly <vilib>:"Digital to Boolean Array.vi"("digital waveform"=w221) -> ()  [unwired: 9 in, 2 out]
          n157 = call-poly <vilib>:"DAQmx Write.vi"("task/channels in"=w281, "auto start"=FALSE, "data"=w221, "error in"=w280) -> ("task out"=w279:refnum<k21>, "error out"=w278:errorcluster)  [unwired: 9 in, 1 out]
          n158 = local write "Digital Waveform Graph"(w221) -> ()
          n159 = local write "Digitaler output"(w221) -> ()
          n160 = call <vilib>:"DAQmx Start Task.vi"("task/channels in"=w279, "error in"=w278) -> ("task out"=w283:refnum<k21>, "error out"=w282:errorcluster)  [unwired: 12 in]
          n161 = flat-sequence {
            tunnel: [w368] -> w290
            tunnel: [w367] -> w289
            tunnel: w286 -> [w366]
            tunnel: w285 -> [w365]
            tunnel: [w364] -> w272
            tunnel: w283 -> [w364]
            tunnel: [w363] -> w271
            tunnel: w282 -> [w363]
            tunnel: [w362] -> w211
            frame #0 {
              n162 = call <vilib>:"DAQmx Start Task.vi"("task/channels in"=w365, "error in"=w366) -> ("task out"=w368:refnum<k21>, "error out"=w367:errorcluster)  [unwired: 12 in]
              n163 = Tick Count (ms)() -> (millisecond timer value=w362:u32)
            }
          }
          n164 = disable-structure shown="Aktiviert" {
            disable-tunnel: w290 -> [w340 _]
            disable-tunnel: w289 -> [w339 _]
            disable-tunnel: [w338 _] -> w215
            disable-tunnel: [w337 _] -> w216
            disable-tunnel: w272 -> [w336 _]
            disable-tunnel: w271 -> [w335 _]
            disable-tunnel: [w334 _] -> w270
            disable-tunnel: [w333 _] -> w210
            disable-tunnel: w211 -> [w332 _]
            disable-tunnel: w203 -> [w331 _]
            frame Enabled {
              n165 = while {
                shift-right: [w358] -> w337
                shift-left: w340 -> [w360]
                shift-right: [w357] -> w338
                shift-left: w339 -> [w359]
                tunnel: w336 -> [w356]
                tunnel: w335 -> [w355]
                tunnel: [w356] -> w334
                tunnel: [w355] -> w333
                tunnel: [w349] -> _
                tunnel: w332 -> [w349]
                tunnel: w331 -> [w346]
                stop <- w351 stop-if-true
                n166 = Tick Count (ms)() -> (millisecond timer value=w347:u32)
                n167 = local read "Stop Boolesch"() -> (w352:bool)
                n168 = Wait (ms)(milliseconds to wait=u32 2 ("Zu wartende ms")) -> ()  [unwired: 1 out]
                n169 = Subtract(x=w347, y=w349) -> (x-y=w342:u32)
                n170 = Subtract(x=w347, y=w346) -> (x-y=w344:u32)
                n171 = call <vilib>:"DAQmx Is Task Done.vi"("task/channels in"=w360, "error in"=w359) -> ("task out"=w358:refnum<k21>, "task done?"=w350:bool, "error out"=w357:errorcluster)  [unwired: 11 in]
                n172 = Unbundle By Name(w357) -> ("status"=w353:bool)
                n173 = Divide(x=w342, y=u32 1000 ("x")) -> (x/y=→"Trial elapsed time":dbl)
                n174 = Divide(x=w344, y=u32 1000 ("x")) -> (x/y=→"Total elapsed time":dbl)
                n175 = Or(x=w353, y=w352) -> (x .or. y?=w361:bool)
                n176 = Or(x=w350, y=w361) -> (x .or. y?=w351:bool)
              }
            }
            frame Disabled {
            }
          }
          n177 = disable-structure shown="Aktiviert" {
            disable-tunnel: w270 -> [w296 _]
            disable-tunnel: [w295 _] -> w214
            disable-tunnel: w210 -> [w294 _]
            disable-tunnel: [w293 _] -> w209
            frame Enabled {
              n178 = call <vilib>:"DAQmx Wait Until Done.vi"("task/channels in"=w296, "error in"=w294) -> ("task out"=w295:refnum<k21>, "error out"=w293:errorcluster)  [unwired: 12 in]
            }
            frame Disabled {
            }
          }
          n179 = flat-sequence {
            tunnel: w216 -> [w315]
            tunnel: w215 -> [w314]
            tunnel: w214 -> [w313]
            tunnel: w209 -> [w312]
            tunnel: w203 -> [w318]
            frame #0 {
              n180 = call <vilib>:"DAQmx Clear Task.vi"("task in"=w315, "error in"=w314) -> ("error out"=w316:errorcluster)  [unwired: 13 in]
              n181 = call <vilib>:"DAQmx Clear Task.vi"("task in"=w313, "error in"=w312) -> ("error out"=w317:errorcluster)  [unwired: 13 in]
              n182 = Merge Errors(w316, w317) -> ()  [unwired: 1 out]
            }
            frame #1 {
              n183 = Tick Count (ms)() -> (millisecond timer value=w319:u32)
              n184 = for {
                N: "Time between trials" -> [_]
                tunnel: w319 -> [w329]
                tunnel: w318 -> [w324]
                stop <- w322 stop-if-true
                w326 = u32 1000 ("Zu wartende ms")
                n185 = Tick Count (ms)() -> (millisecond timer value=w323:u32)
                n186 = Subtract(x=w323, y=w329) -> (x-y=w330:u32)
                n187 = Subtract(x=w323, y=w324) -> (x-y=w327:u32)
                n188 = local read "Stop Boolesch"() -> (w322:bool)
                n189 = Divide(x=w330, y=w326) -> (x/y=→"Pause elapsed time":dbl)
                n190 = Divide(x=w327, y=w326) -> (x/y=w325:dbl)
                n191 = local write "Total elapsed time"(w325) -> ()
                n192 = Wait (ms)(milliseconds to wait=w326) -> ()  [unwired: 1 out]
              }
              "In between trials" <- TRUE ("In between trials")
            }
          }
          n193 = local read "Stop Boolesch"() -> (w217:bool)
          "Current Valve" <- w207
          "Current list index" <- w213
        }
        n194 = local write "Experiment running"(TRUE ("Experiment running")) -> ()
        "State" <- w199
      }
      frame "Stop" {
        n195 = local write "State"(w369) -> ()
        n196 = flat-sequence {
          frame #0 {
            # "Stop-all to zero"
            # "all lines also trigger line"
            n197 = call-poly <vilib>:"DAQmx Write.vi"("task/channels in"="/Dev2/port0/line17:25" ("string"), "data"=bool[] [FALSE, FALSE, FALSE, FALSE, FALSE, FALSE, FALSE, FALSE, FALSE]) -> ("task out"=w377:refnum<k21>, "error out"=w372:errorcluster)  [unwired: 11 in, 1 out]
            n198 = call <vilib>:"DAQmx Start Task.vi"("task/channels in"=w377, "error in"=w372) -> ("task out"=w376:refnum<k21>, "error out"=w374:errorcluster)  [unwired: 12 in]
            n199 = call <vilib>:"DAQmx Wait Until Done.vi"("task/channels in"=w376, "error in"=w374) -> ("task out"=w375:refnum<k21>, "error out"=w373:errorcluster)  [unwired: 12 in]
            n200 = call <vilib>:"DAQmx Clear Task.vi"("task in"=w375, "error in"=w373) -> ()  [unwired: 13 in, 1 out]
          }
          frame #1 {
            w383 = T2."Enabled" ("Deaktiviert")
            n201 = property on="Select experiment" class="TabCtl (strict)"() -> ("Pages"=w382:refnum<vi>[])  [unwired: 2 in, 2 out]
            n202 = property on="Valve order list" class="Arr (strict)"("DisabledEnum"=T2."Enabled" ("Deaktiviert")) -> ()  [unwired: 2 in, 2 out]
            n203 = for {
              tunnel: w382 -> [w384] mode=indexing
              n204 = property class="Page"(reference=w384, "PageEnb"=T3."Page Enabled" ("Aktiv-Status der Seite")) -> ()  [unwired: 1 in, 2 out]
            }
            n205 = property on="Start trial series" class="Bool"("DisabledEnum"=w383) -> ()  [unwired: 2 in, 2 out]
            n206 = property on="Start single trial" class="Bool"("DisabledEnum"=w383) -> ()  [unwired: 2 in, 2 out]
            "Experiment running" <- FALSE ("Experiment running")
          }
        }
        n207 = local read "Stop Boolesch"() -> (w371:bool)
      }
    }
  }
  n208 = while {
    tunnel: w4 -> [w387]
    stop <- w386 stop-if-true
    n209 = event shown="[2] \"Stopp\": Value Change" {
      selector: _ -> [_ _ _ _]
      dyn-events: _ -> [_ _ _ _]
      timeout: _ -> [_ _ _ _]
      tunnel: w387 -> [_ w388 w397 w403]
      event Timeout {
        n210 = event-data() -> ()  [unwired: 1 in, 3 out]
      }
      event "Start single trial": Value Change {
        n211 = event-data() -> ()  [unwired: 1 in, 6 out]
        n212 = case shown="True" "Start single trial" {
          tunnel: w388 -> [_ w396]
          frame False {
          }
          frame True {
            n213 = property on="Start single trial" class="Bool"("DisabledEnum"=T2."Disabled and Grayed Out" ("Deaktiviert")) -> ()  [unwired: 2 in, 2 out]
            n214 = Enqueue Element(queue=w396, element=StatesEnum."Start Trial" ("Enum")) -> ()  [unwired: 2 in, 3 out]
            n215 = property on="Select experiment" class="TabCtl (strict)"() -> ("Pages"=w392:refnum<vi>[])  [unwired: 2 in, 2 out]
            n216 = Index Array(array=w392, index=1 ("Index")) -> (element=w393:refnum<vi>)
            n217 = property class="Page"(reference=w393, "PageEnb"=T3."Page Disabled & Grayed" ("Aktiv-Status der Seite")) -> ()  [unwired: 1 in, 2 out]
          }
        }
      }
      event "Stopp": Value Change {
        n218 = event-data() -> ()  [unwired: 1 in, 6 out]
        n219 = case shown="True" "Stopp" {
          tunnel: w397 -> [_ w401]
          frame False {
          }
          frame True {
            n220 = Enqueue Element(queue=w401, element=StatesEnum."Stop" ("Enum")) -> ()  [unwired: 2 in, 3 out]
            "Stop Boolesch" <- TRUE ("Stop Boolesch")
          }
        }
      }
      event "Start trial series": Value Change {
        n221 = event-data() -> ()  [unwired: 1 in, 6 out]
        n222 = case shown="True" "Start trial series" {
          tunnel: w403 -> [_ w410]
          frame False {
          }
          frame True {
            n223 = property on="Start trial series" class="Bool"("DisabledEnum"=T2."Disabled and Grayed Out" ("Deaktiviert")) -> ()  [unwired: 2 in, 2 out]
            n224 = Enqueue Element(queue=w410, element=StatesEnum."Start trial series" ("Enum")) -> ()  [unwired: 2 in, 3 out]
            n225 = property on="Select experiment" class="TabCtl (strict)"() -> ("Pages"=w406:refnum<vi>[])  [unwired: 2 in, 2 out]
            n226 = Index Array(array=w406, index=0 ("Index")) -> (element=w407:refnum<vi>)
            n227 = property class="Page"(reference=w407, "PageEnb"=T3."Page Disabled & Grayed" ("Aktiv-Status der Seite")) -> ()  [unwired: 1 in, 2 out]
          }
        }
      }
    }
    n228 = local read "Stop Boolesch"() -> (w386:bool)
  }
  n229 = Release Queue(queue=w3) -> ()  [unwired: 2 in, 3 out]
